vi "Compute DistanceToTarget.vi"(8 "Y Image Resolution":i32, 9 "X Image Resolution":i32, 10 "Vertical Strip":T1) -> (2 "Target Center (-1 to 1)":cluster{"X":dbl, "Y":dbl}, 3 "Distance (ft)":dbl)   [LabVIEW 2013]
doc: "Using the camera lens information and the real world size of the target, use trig and ratios to determine the distance to the target. Also returns the location relative to the image center in a (-1 , 1) coordinate system that may be useful for steering the robot."
panel:
  # "Axis 206\nAxis M1011\nAxis M1013"
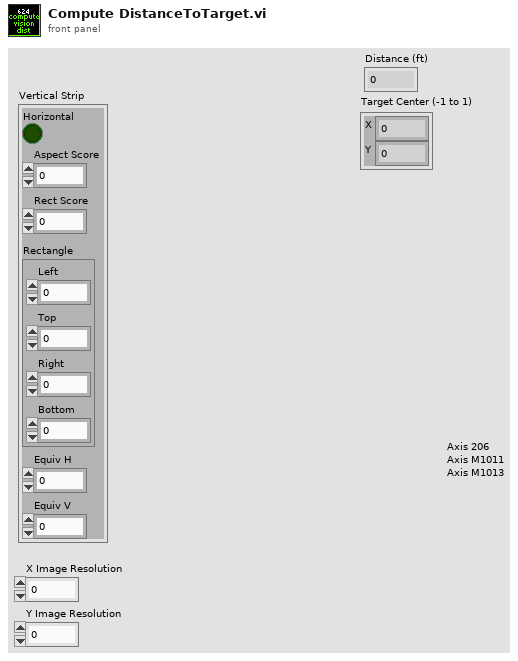
[diagram p1: front panel]
types:
  T1 = cluster{"Horizontal":bool, "Aspect Score":dbl, "Rect Score":dbl, "Rectangle":cluster{"Left":dbl, "Top":dbl, "Right":dbl, "Bottom":dbl}, "Equiv H":dbl, "Equiv V":dbl}
  T2 = cluster{"X Image Resolution":i32, "Y Image Resolution":i32}
  T3 = cluster{"X Image Resolution":dbl, "Y Image Resolution":dbl}
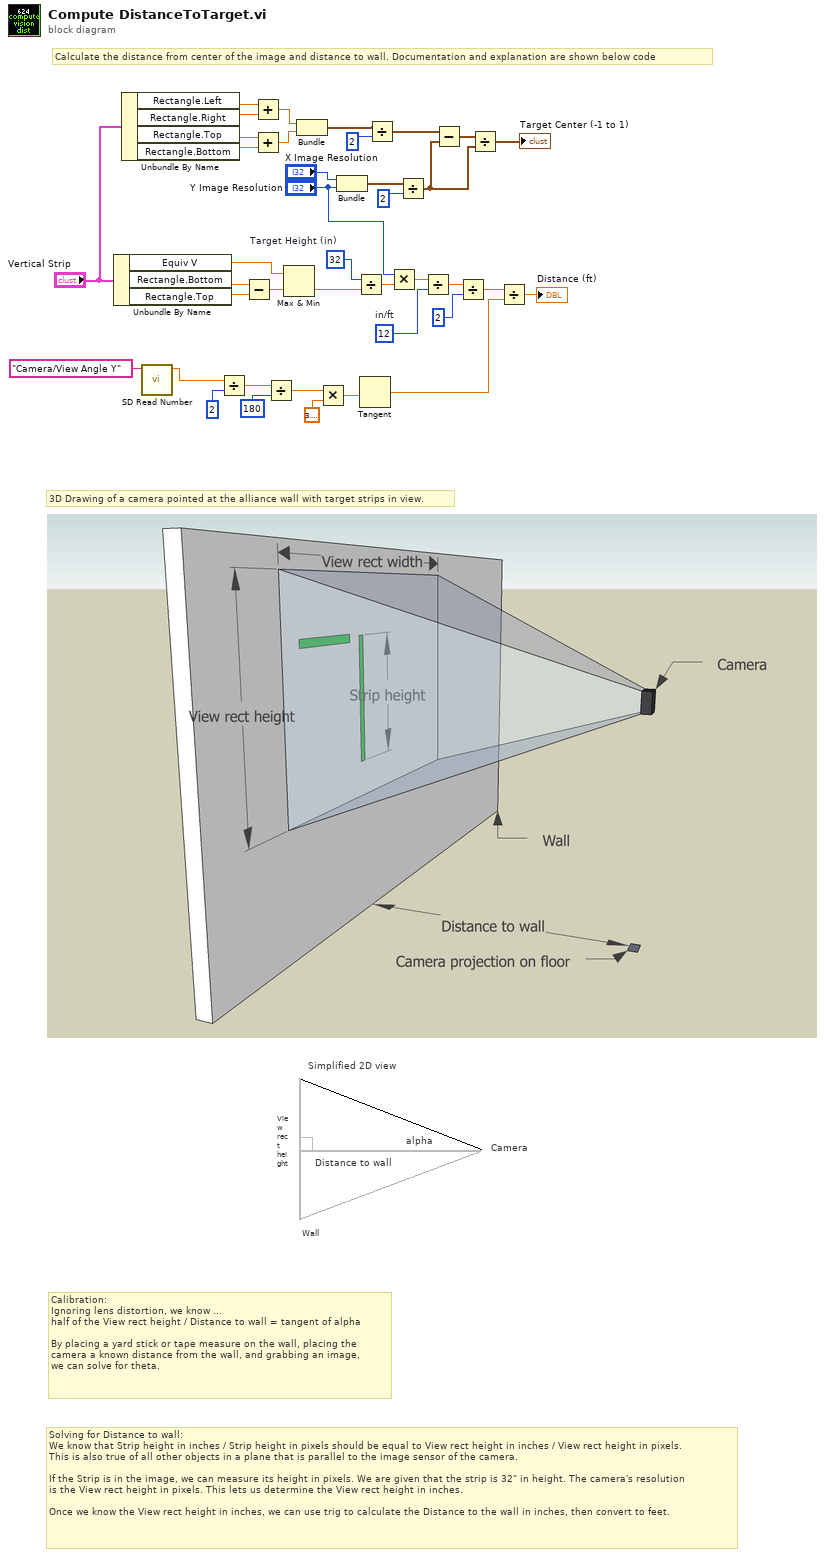
[diagram p0: block diagram]
diagram:
  w8 = 12  # in/ft
  w13 = 32  # Target Height (in)
  # "Wall"
  # "Camera"
  # "Simplified 2D view"
  # "Solving for Distance to wall:\nWe know that Strip height in inches / Strip height in pixels should be equal to View rect height in inches / View rect height in pixels.\nThis is also true of all other objects in a plane that is parallel to the image sensor of the camera.\n\nIf the Strip is in the image, we can measure its height in pixels. We are given that the strip is 32\" in height. The camera's resolution\nis the View rect height in pixels. This lets us determine the View rect height in inches.\n\nOnce we know the View rect height in inches, we can use trig to calculate the Distance to the wall in inches, then convert to feet."
  # "3D Drawing of a camera pointed at the alliance wall with target strips in view."
  # "Distance to wall"
  # "View rect height"
  # "alpha"
  # "Calibration:\nIgnoring lens distortion, we know ...\nhalf of the View rect height / Distance to wall = tangent of alpha\n\nBy placing a yard stick or tape measure on the wall, placing the\ncamera a known distance from the wall, and grabbing an image,\nwe can solve for theta."
  # "Calculate the distance from center of the image and distance to wall. Documentation and explanation are shown below code"
  n1 = Unbundle By Name("Vertical Strip") -> ("Equiv V"=w16:dbl, "Rectangle.Bottom"=w33:dbl, "Rectangle.Top"=w32:dbl)
  n2 = Unbundle By Name("Vertical Strip") -> ("Rectangle.Left"=w27:dbl, "Rectangle.Right"=w28:dbl, "Rectangle.Top"=w30:dbl, "Rectangle.Bottom"=w29:dbl)
  n3 = call <vilib>:"SD Read Number.vi"("Name"="Camera/View Angle Y") -> ("Numeric"=w2:dbl)  [unwired: 8 in, 2 out]
  n4 = Divide(x=w2, y=2) -> (x/y=w36:dbl)
  n5 = Subtract(x=w33, y=w32) -> (x-y=w15:dbl)
  n6 = Add(x=w27, y=w28) -> (x+y=w25:dbl)
  n7 = Add(x=w30, y=w29) -> (x+y=w24:dbl)
  n8 = Divide(x=w36, y=180) -> (x/y=w35:dbl)
  n9 = Max & Min(x=w16, y=w15) -> (min(x,y)=w12:dbl)  [unwired: 1 out]
  n10 = Bundle(w25, w24) -> (w21:cluster{dbl, dbl})  [unwired: 1 in]
  n11 = Multiply(x=w35, y=3.141592653589793) -> (x*y=w37:dbl)
  n12 = Bundle("X Image Resolution"="X Image Resolution", "Y Image Resolution"="Y Image Resolution") -> (w23:T2)  [unwired: 1 in]
  n13 = Divide(x=w13, y=w12) -> (x/y=w11:dbl)
  n14 = Tangent(1:w37) -> (0:w4:dbl)
  n15 = Divide(x=w21, y=2) -> (x/y=w20:cluster{dbl, dbl})
  n16 = Multiply(x="Y Image Resolution", y=w11) -> (x*y=w9:dbl)
  n17 = Divide(x=w23, y=2) -> (x/y=w18:T3)
  n18 = Divide(x=w9, y=w8) -> (x/y=w7:dbl)
  n19 = Subtract(x=w20, y=w18) -> (x-y=w19:cluster{dbl, dbl})
  n20 = Divide(x=w7, y=2) -> (x/y=w5:dbl)
  n21 = Divide(x=w19, y=w18) -> (x/y=→"Target Center (-1 to 1)":cluster{dbl, dbl})
  n22 = Divide(x=w5, y=w4) -> (x/y=→"Distance (ft)":dbl)
